vi "PWM.Measure.Analog.vi"(10 "PWM":fxp<+/-,32,8>, 11 "Settings":T3={"ACTIVE EDGE"=TRUE, "TIMEOUT"=40000000, "THRESHOLD"=50.0}) -> (2 "Update?":bool, 3 "Measurement":T1)   [LabVIEW 2015, in "Speciality FPGA IO.lvlib"]
uses:
  Speciality FPGA IO.lvlib
  Types/PWM.Measure.Analog.Settings.ctl
  Types/PWM.Measure.Analog.Internal.ctl
  Types/PWM.Measure.Analog.Measurement.ctl
  <vilib>/rvi/Emulation/niFpgaSctlEmulationGetInTimedLoop.vi
  <vilib>/rvi/Emulation/niFpgaProcessEmulError.vi
panel:
  out "Local.State":bool
  out "Local.Data":T2
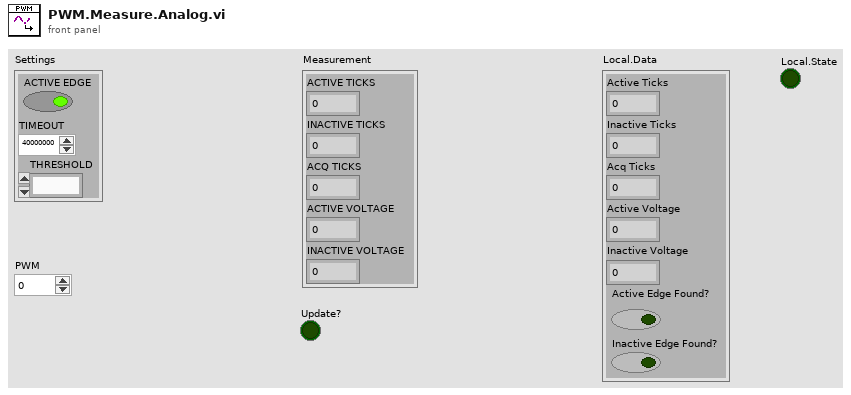
[diagram p1: front panel]
types:
  T1 = typedef "Speciality FPGA IO.lvlib/PWM.Measure.Analog.Measurement.ctl" = cluster{"ACTIVE TICKS":u32, "INACTIVE TICKS":u32, "ACQ TICKS":u32, "ACTIVE VOLTAGE":fxp<+/-,32,8>, "INACTIVE VOLTAGE":fxp<+/-,32,8>}
  T2 = typedef "Speciality FPGA IO.lvlib/PWM.Measure.Analog.Internal.ctl" = cluster{"Active Ticks":u32, "Inactive Ticks":u32, "Acq Ticks":u32, "Active Voltage":fxp<+/-,32,8>, "Inactive Voltage":fxp<+/-,32,8>, "Active Edge Found?":bool, "Inactive Edge Found?":bool}
  T3 = typedef "Speciality FPGA IO.lvlib/PWM.Measure.Analog.Settings.ctl" = cluster{"ACTIVE EDGE":bool, "TIMEOUT":u32, "THRESHOLD":fxp<+/-,32,8>}
  T4 = enum8{"Initialize", "Wait on Active Edge", "Wait on Inactive Edge"}
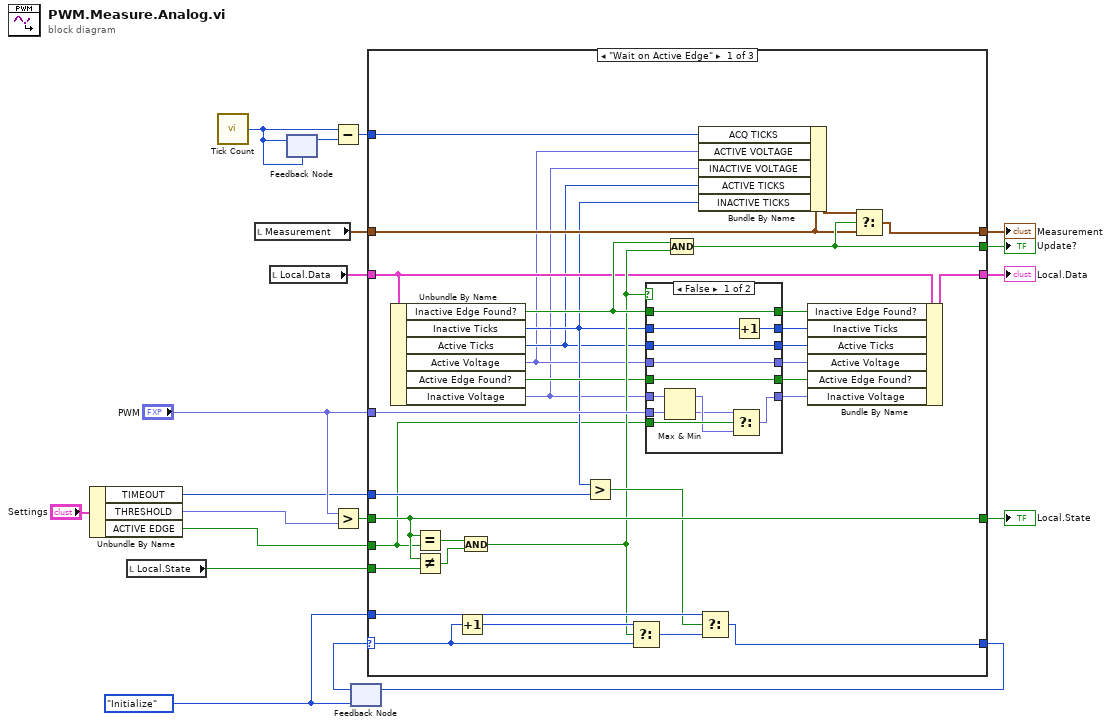
[diagram p0: block diagram]
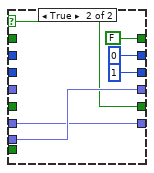
[diagram p2: hidden frame]
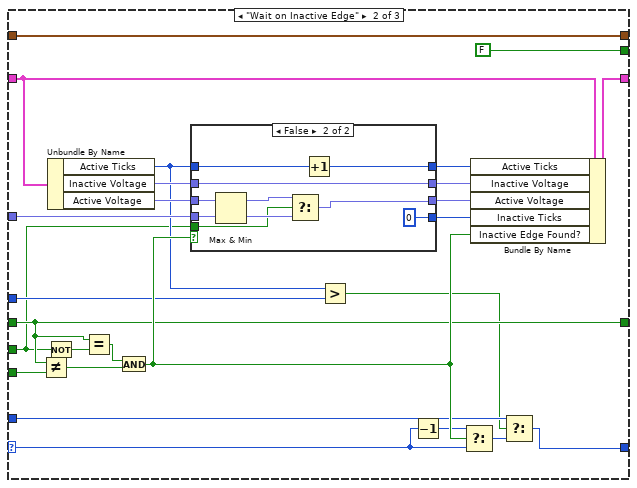
[diagram p3: hidden frame]
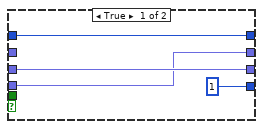
[diagram p4: hidden frame]
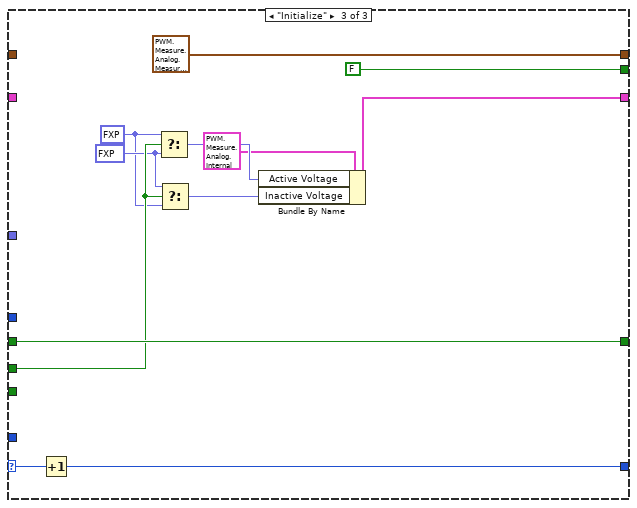
[diagram p5: hidden frame]
diagram:
  w8 = T4."Initialize"
  n1 = Unbundle By Name("Settings") -> ("TIMEOUT"=w2:u32, "THRESHOLD"=w1:fxp<+/-,32,8>, "ACTIVE EDGE"=w14:bool)
  n2 = local read "Local.State"() -> (w12:bool)
  n3 = call "Tick Count"() -> ("Tick Count(Ticks)"=w5:u32)
  n4 = local read "Measurement"() -> (w10:T1)
  n5 = local read "Local.Data"() -> (w16:T2)
  n6 = feedback-in #1(w5) -> ()
  n7 = feedback #1(w5) -> (w6:u32)
  n8 = Subtract(x=w5, y=w6) -> (x-y=w4:u32)
  n9 = Greater?(x="PWM", y=w1) -> (0:w15:bool)
  n10 = feedback #2(w8) -> (w18:T4)
  n11 = case shown="\"Wait on Active Edge\"" w18 {
    selector: w18 -> [w51 w80 w122]
    tunnel: [w49 w94 w114] -> w19
    tunnel: [w33 w73 w121] -> w17
    tunnel: w16 -> [w28 w93 _]
    tunnel: w15 -> [w41 w82 w120]
    tunnel: w14 -> [w20 w71 w119]
    tunnel: [w41 w82 w120] -> w13
    tunnel: w12 -> [w52 w96 _]
    tunnel: "PWM" -> [w43 w91 _]
    tunnel: [w44 w88 T1 {"ACTIVE TICKS"=0, "INACTIVE TICKS"=0, "ACQ TICKS"=0, "ACTIVE VOLTAGE"=0.0, "INACTIVE VOLTAGE"=0.0} ("Cached.Data")] -> w3
    tunnel: w10 -> [w25 w88 _]
    tunnel: w2 -> [w37 w77 _]
    tunnel: w8 -> [w36 w76 _]
    tunnel: [w32 FALSE FALSE] -> w7
    tunnel: w4 -> [w26 _ _]
    frame "Wait on Active Edge" {
      n12 = Unbundle By Name(w28) -> ("Inactive Edge Found?"=w45:bool, "Inactive Ticks"=w24:u32, "Active Ticks"=w23:u32, "Active Voltage"=w22:fxp<+/-,32,8>, "Active Edge Found?"=w29:bool, "Inactive Voltage"=w21:fxp<+/-,32,8>)
      n13 = Equal?(x=w41, y=w20) -> (x = y?=w40:bool)
      n14 = Not Equal?(x=w41, y=w52) -> (x != y?=w39:bool)
      n15 = Increment(x=w51) -> (x+1=w50:T4)
      n16 = And(x=w40, y=w39) -> (x .and. y?=w31:bool)
      n17 = Greater?(x=w24, y=w37) -> (0:w35:bool)
      n18 = Select(t=w50, s=w31, f=w51) -> (s? t:f=w34:T4)
      n19 = case shown="False" w31 {
        selector: w31 -> [_ w65]
        tunnel: [w53 w67] -> w48
        tunnel: [w63 u32 0 ("Inactive time")] -> w47
        tunnel: w24 -> [w64 _]
        tunnel: w21 -> [w62 w67]
        tunnel: w45 -> [w61 _]
        tunnel: [w61 FALSE ("Inactive Edge Found?")] -> w46
        tunnel: w43 -> [w60 w68]
        tunnel: [w59 w68] -> w42
        tunnel: w22 -> [w59 _]
        tunnel: [w58 u32 1 ("t")] -> w38
        tunnel: w23 -> [w58 _]
        tunnel: [w57 w65] -> w30
        tunnel: w29 -> [w57 _]
        tunnel: w20 -> [w56 _]
        frame False {
          n20 = Max & Min(x=w62, y=w60) -> (max(x,y)=w55:fxp<+/-,32,8>, min(x,y)=w54:fxp<+/-,32,8>)
          n21 = Select(t=w54, s=w56, f=w55) -> (s? t:f=w53:fxp<+/-,32,8>)
          n22 = Increment(x=w64) -> (x+1=w63:u32)
        }
        frame True {
        }
      }
      n23 = Compound Arithmetic op=AND(w45, w31) -> (w32:bool)
      n24 = Bundle By Name(cluster=w25, "ACQ TICKS"=w26, "ACTIVE VOLTAGE"=w22, "INACTIVE VOLTAGE"=w21, "ACTIVE TICKS"=w23, "INACTIVE TICKS"=w24) -> (w27:T1)
      n25 = Select(t=w36, s=w35, f=w34) -> (s? t:f=w33:T4)
      n26 = Bundle By Name(cluster=w28, "Inactive Edge Found?"=w46, "Inactive Ticks"=w47, "Active Ticks"=w38, "Active Voltage"=w42, "Active Edge Found?"=w30, "Inactive Voltage"=w48) -> (w49:T2)
      n27 = Select(t=w27, s=w32, f=w25) -> (s? t:f=w44:T1)
    }
    frame "Wait on Inactive Edge" {
      n28 = Not Equal?(x=w82, y=w96) -> (x != y?=w95:bool)
      n29 = Not(x=w71) -> (.not. x?=w83:bool)
      n30 = Unbundle By Name(w93) -> ("Active Ticks"=w78:u32, "Inactive Voltage"=w86:fxp<+/-,32,8>, "Active Voltage"=w92:fxp<+/-,32,8>)
      n31 = Equal?(x=w82, y=w83) -> (x = y?=w81:bool)
      n32 = And(x=w81, y=w95) -> (x .and. y?=w84:bool)
      n33 = case shown="False" w84 {
        tunnel: w92 -> [w99 w110]
        tunnel: w91 -> [w98 w109]
        tunnel: [w99 w102] -> w90
        tunnel: w78 -> [w100 w108]
        tunnel: [w100 w107] -> w89
        tunnel: [w98 w106] -> w87
        tunnel: w86 -> [_ w106]
        tunnel: [u32 1 ("t") u32 0 ("t")] -> w85
        tunnel: w71 -> [_ w101]
        frame True {
        }
        frame False {
          n34 = Max & Min(x=w110, y=w109) -> (max(x,y)=w103:fxp<+/-,32,8>, min(x,y)=w104:fxp<+/-,32,8>)
          n35 = Select(t=w103, s=w101, f=w104) -> (s? t:f=w102:fxp<+/-,32,8>)
          n36 = Increment(x=w108) -> (x+1=w107:u32)
        }
      }
      n37 = Greater?(x=w78, y=w77) -> (0:w75:bool)
      n38 = Decrement(x=w80) -> (x-1=w79:T4)
      n39 = Select(t=w79, s=w84, f=w80) -> (s? t:f=w74:T4)
      n40 = Bundle By Name(cluster=w93, "Active Ticks"=w89, "Inactive Voltage"=w87, "Active Voltage"=w90, "Inactive Ticks"=w85, "Inactive Edge Found?"=w84) -> (w94:T2)
      n41 = Select(t=w76, s=w75, f=w74) -> (s? t:f=w73:T4)
    }
    frame "Initialize" {
      w117 = fxp<+/-,32,8> -128.0 ("Active Voltage")
      w116 = fxp<+/-,32,8> 127.99998474121094 ("Active Voltage")
      n42 = Increment(x=w122) -> (x+1=w121:T4)
      n43 = Select(t=w116, s=w119, f=w117) -> (s? t:f=w118:fxp<+/-,32,8>)
      n44 = Select(t=w117, s=w119, f=w116) -> (s? t:f=w115:fxp<+/-,32,8>)
      n45 = Bundle By Name(cluster=T2 {"Active Ticks"=0, "Inactive Ticks"=0, "Acq Ticks"=0, "Active Voltage"=0.0, "Inactive Voltage"=0.0, "Active Edge Found?"=FALSE, "Inactive Edge Found?"=FALSE} ("Result"), "Active Voltage"=w118, "Inactive Voltage"=w115) -> (w114:T2)
    }
  }
  "Local.Data" <- w19
  "Local.State" <- w13
  "Measurement" <- w3
  "Update?" <- w7
  n46 = feedback-in #2(w17) -> ()
